vi "Read Samples.vi"(8 "error in (no error)":errorcluster, 11 "Metric in":refnum<class "Metric.lvclass">) -> (0 "error out":errorcluster, 2 "Samples":refnum<class "Sample.lvclass">[](array[class]), 3 "Metric out":refnum<class "Metric.lvclass">)   [LabVIEW 2020, in "Metrics.lvlib" / "Metric.lvclass"]
uses:
  Metric.lvclass
  sample/Sample.lvclass
  Metric.lvclass/Metric.ctl
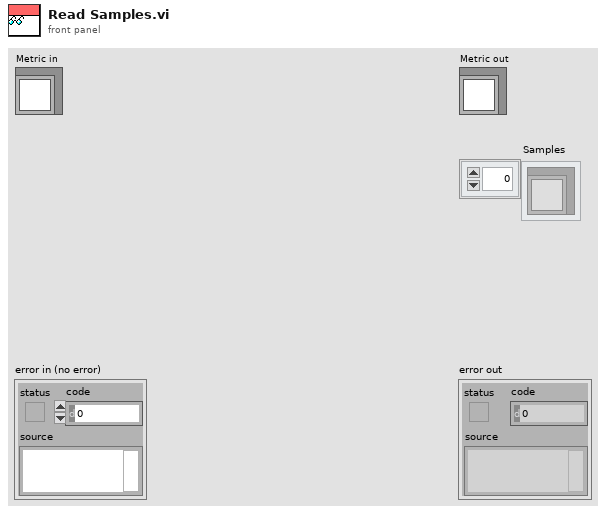
[diagram p1: front panel]
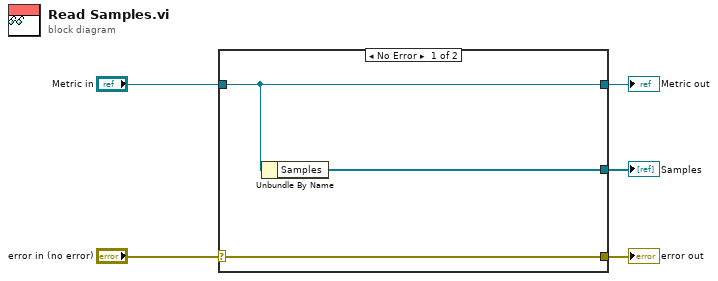
[diagram p0: block diagram]
diagram:
  n1 = case shown="No Error" "error in (no error)" {
    selector: "error in (no error)" -> [w8 w9]
    tunnel: [w8 w9] -> w4
    tunnel: [w7 w10] -> w2
    tunnel: "Metric in" -> [w7 w10]
    tunnel: [w6 _] -> w1
    frame No Error {
      n2 = Unbundle By Name(w7) -> ("Samples"=w6:refnum<class "Sample.lvclass">[])
    }
    frame Error {
    }
  }
  "error out" <- w4
  "Metric out" <- w2
  "Samples" <- w1
